vi "Set Initialized Fields.vi"(8 "error in (no error)":errorcluster, 10 "Initialized Fields":set{string}(c389), 11 "Object Type in":refnum<class "Object Type Base.lvclass">) -> (0 "error out":errorcluster, 3 "Object Type out":refnum<class "Object Type Base.lvclass">)   [LabVIEW 2024, in "EDS.lvlib" / "Object Type Base.lvclass"]
uses:
  Object Type Base.lvclass
  Object Type Base.lvclass/Object Type Base.ctl
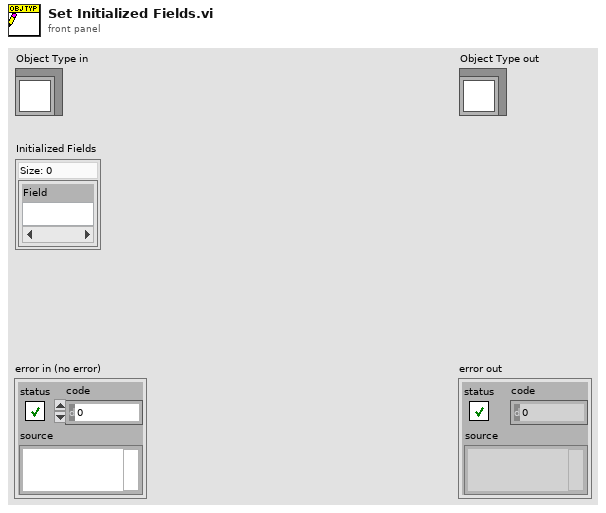
[diagram p1: front panel]
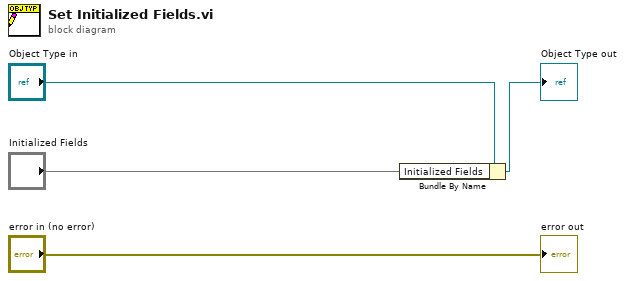
[diagram p0: block diagram]
diagram:
  n1 = Bundle By Name(cluster="Object Type in", "Initialized Fields"="Initialized Fields") -> (→"Object Type out":refnum<class "Object Type Base.lvclass">)
  "error out" <- "error in (no error)"
